vi "LJM logger apply formula in tc.vi"(1 "Input Values":dbl[][](array[numeric]) format="%.2f", 2 "Variables Input":string[](array[string])=["v1", "v2", "v3", "v4"], 3 "formula":string, 4 "error in (no error)":errorcluster) -> (5 "Output Values":dbl[](array[numeric]) format="%.2f", 6 "error out":errorcluster)   [LabVIEW 2026]
doc: "Similar to the Formula Node function, but with variables that can be entered on the front panel."
uses:
  <vilib>/gmath/NI_Gmath.lvlib
panel:
  in  "Variables Output":string[](array[string])=["y"]
  # "Input = v\nOutput = y"
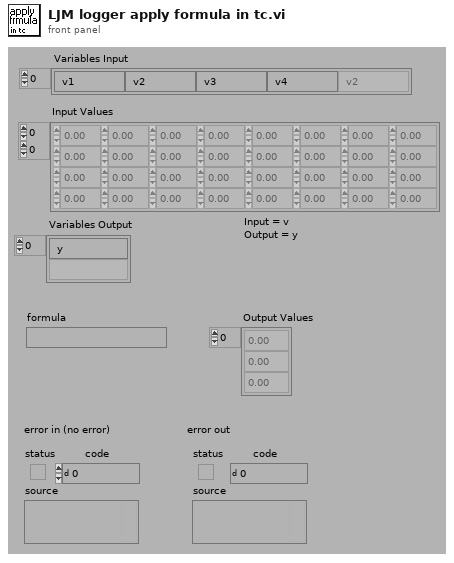
[diagram p1: front panel]
types:
  T1 = cluster{"Y Values":dbl[][], "Tables":i32[][][], "Variables input decode":i32[], "Variables output decode":i32[]}
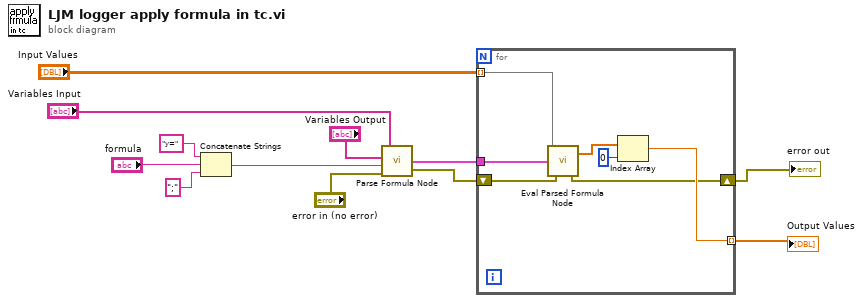
[diagram p0: block diagram]
diagram:
  n1 = Concatenate Strings("y=" ("Substring"), "formula", ";" ("Substring")) -> (w1:string)
  n2 = call <vilib>:"Parse Formula Node.vi"("error in (no error)"="error in (no error)", "formula"=w1, "Variables Output"="Variables Output", "Variables Input"="Variables Input") -> ("error out"=w11:errorcluster, "Parsed Formula Node"=w10:T1)
  n3 = for {
    tunnel: "Input Values" -> [w13] mode=indexing
    tunnel: w10 -> [w19]
    tunnel: [w16] -> w9 mode=indexing
    shift-right: [w14] -> w12
    shift-left: w11 -> [w15]
    n4 = call <vilib>:"Eval Parsed Formula Node.vi"("error in (no error)"=w15, "Parsed Formula Node"=w19, "Input Values"=w13) -> ("error out"=w14:errorcluster, "Output Values"=w18:dbl[])
    n5 = Index Array(array=w18, index=0 ("Index")) -> (element=w16:dbl)
  }
  "Output Values" <- w9
  "error out" <- w12
